vi "Dictionary.Add File and Notes.vi"(2 "Notes":string, 3 "Path":path) -> (1 "Dictionary":T1[](array[typedef]))   [LabVIEW 2019, in "Conversion.lvclass"]
uses:
  Conversion.lvclass
  Data/Typedefs/Dictionary--cluster.ctl
  Data/Data.lvclass
panel:
  out "stripped path":path
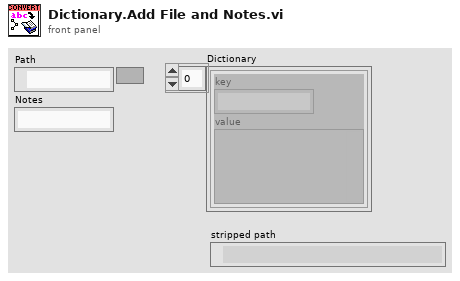
[diagram p1: front panel]
types:
  T1 = typedef "Data.lvclass/Dictionary--cluster.ctl" = cluster{"key":string, "value":variant}
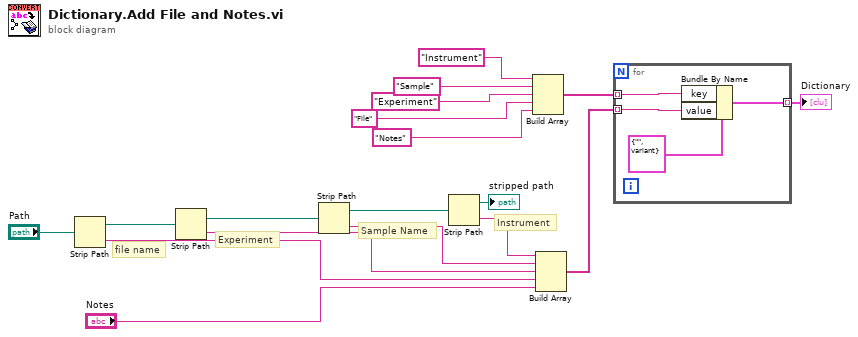
[diagram p0: block diagram]
diagram:
  # "Instrument"
  # "Sample Name"
  # "Experiment"
  # "file name"
  n1 = Strip Path(path="Path") -> (stripped path=w6:path, name=w12:string)
  n2 = Strip Path(path=w6) -> (stripped path=w7:path, name=w10:string)
  n3 = Strip Path(path=w7) -> (stripped path=w8:path, name=w11:string)
  n4 = Strip Path(path=w8) -> (stripped path=→"stripped path":path, name=w9:string)
  n5 = Build Array("Instrument", "Sample", "Experiment", "File", "Notes") -> (w3:string[])
  n6 = Build Array(w9, w11, w10, w12, "Notes") -> (w4:string[])
  n7 = for {
    tunnel: w4 -> [w22] mode=indexing
    tunnel: w3 -> [w21] mode=indexing
    tunnel: [w19] -> w2 mode=indexing
    n8 = Bundle By Name(cluster=T1 {"key"="", "value"=variant} ("key-value"), "key"=w21, "value"=w22) -> (w19:T1)
  }
  "Dictionary" <- w2
